vi "Rinocloud_real-time_monitoring.vi"() -> ()   [LabVIEW 2011, in "Rinocloud Library.lvlib"]
uses:
  Rinocloud Library.lvlib
  Rinocloud_global_variable.vi
  Rinocloud API endpoint VIs/API_endpoint_subVIs/Rinocloud_get_metadata_field_value_subVIs/get_string_value.vi
  Rinocloud API endpoint VIs/API_endpoint_subVIs/Rinocloud_get_metadata_field_value_subVIs/get_numeric_value.vi
panel:
  out "Local status:":string="OFF"
  in  "Toggle":bool
  out "Sending...":bool
  out "System Waveform Graph":dbl[](graph)
  out "Data chunk":string
  in  "Record name":string
  in  "create empty":bool
  in  "Request period (s)":dbl=1.0 format="%#.2f"
  out "Remote status:":string="OFF"
  in  "stop":bool
  out "Parent folder:":string
  # "Request period and measurement status\ncan be set remotely by\n{\"period\":<value in s>, \"status\":\"on<or off>\"}\n\nLocal changes of period or/and status are \nupdated immediatelly on Rinocloud."
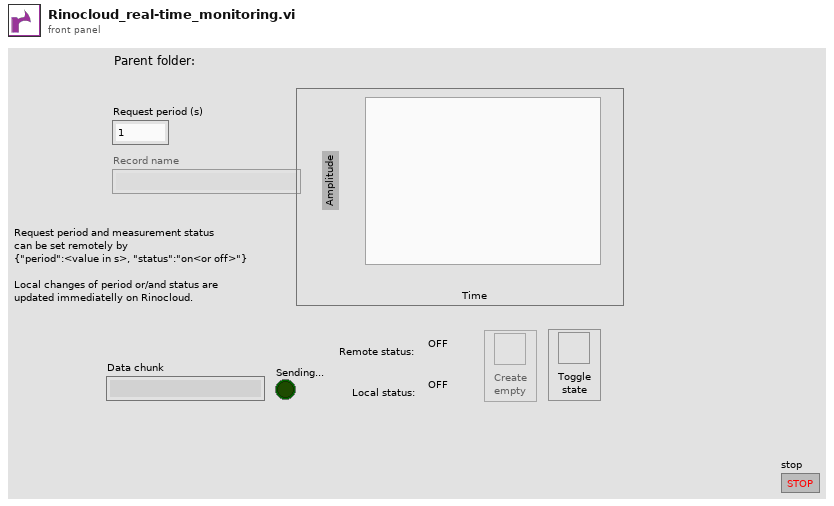
[diagram p1: front panel]
types:
  T1 = cluster{"Record ID":string, "Status":string, "Record name":string, "Parent ID":string, "Request period (s)":dbl, "Sending...":bool, "Parent folder":string, "HTTP resp body":string, "Data chunk":string, "error out":errorcluster, "error in (no error)":errorcluster, "x":dbl, "y array":dbl[], "y":dbl}
  T2 = enum16{"initialize", "create empty", "append", "wait for event", "start append", "generate data"}
  T3 = enum8{"Enabled", "Disabled", "Disabled and Grayed Out"}
  T4 = enum16{"initialize", "create empty", "append", "wait for event"}
  T5 = cluster{"Attribute":string, "Value":string, "Data type":enum16{"Numeric", "String", "1D array of strings", "1D array of doubles", "Data JSON string", "<null>"}}
  T6 = enum16{"Numeric", "String", "1D array of strings", "1D array of doubles", "Data JSON string", "<null>"}
  T7 = cluster{"Attribute":string, "Value":string, "Data type":enum16{"Numeric", "String", "1D array of strings", "1D array of doubles", "Data JSON string", "<null>"}}[]
  T8 = cluster{"headers":string, "body":string, "ID":string, "Saved":bool}
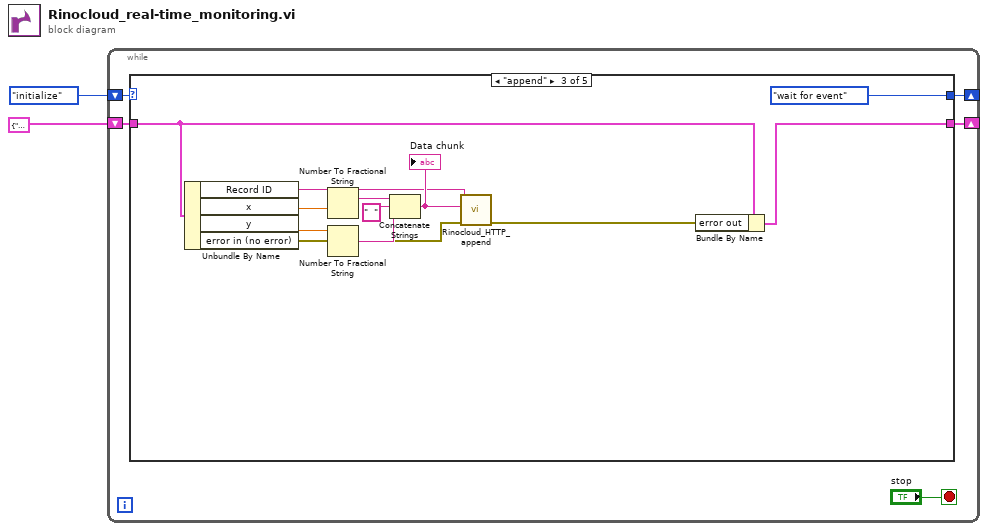
[diagram p0: block diagram]
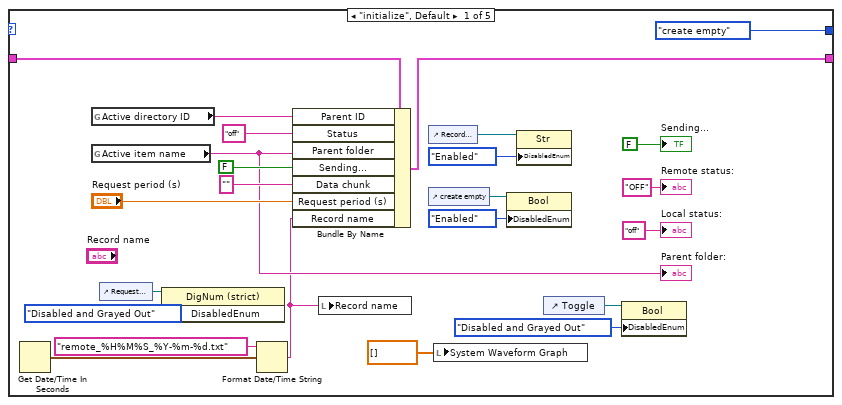
[diagram p2: hidden frame]
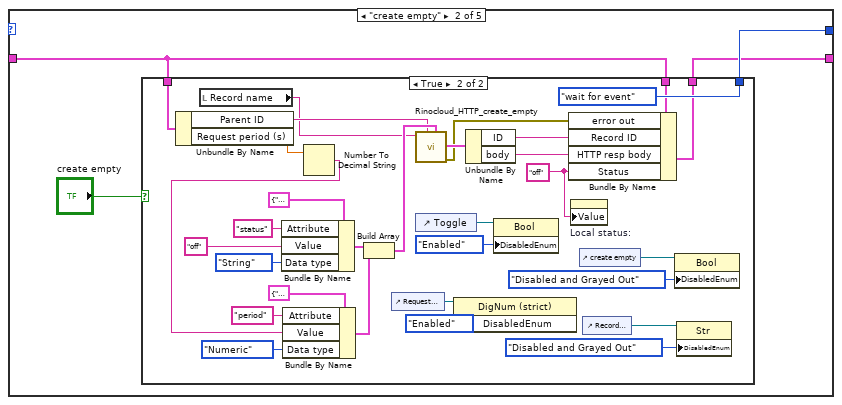
[diagram p3: hidden frame]
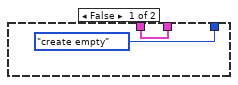
[diagram p4: hidden frame]
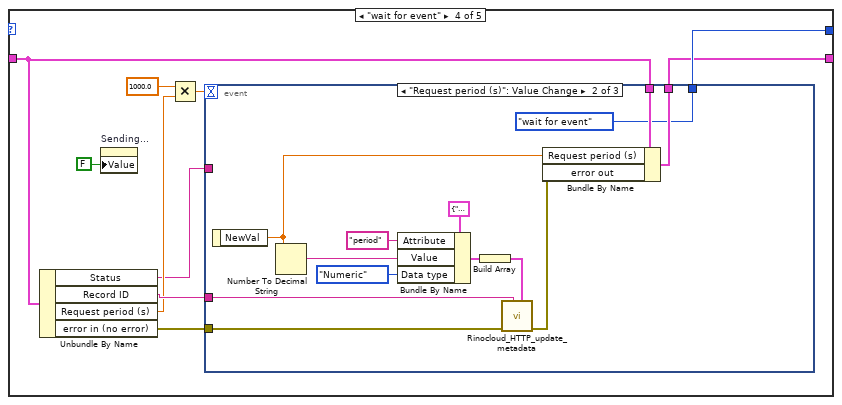
[diagram p5: hidden frame]
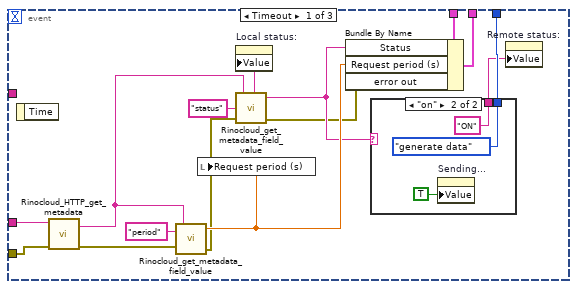
[diagram p6: hidden frame]
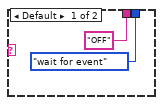
[diagram p7: hidden frame]
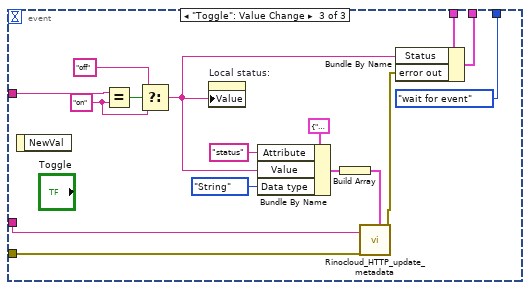
[diagram p8: hidden frame]
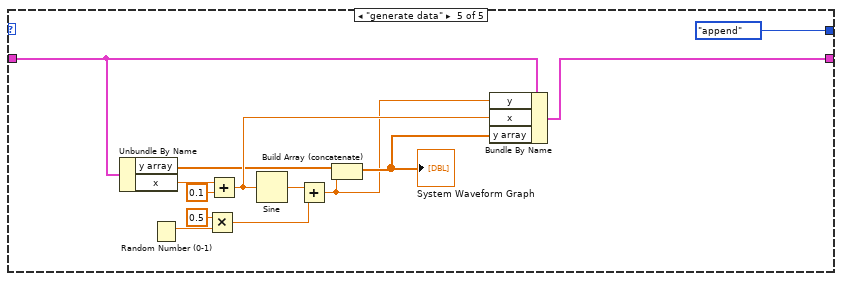
[diagram p9: hidden frame]
diagram:
  n1 = while {
    shift-right: [w3] -> _
    shift-left: T2."initialize" -> [w4]
    shift-right: [w5] -> _
    shift-left: T1 {"Record ID"="", "Status"="", "Record name"="", "Parent ID"="", "Request period (s)"=1.0, "Sending..."=FALSE, "Parent folder"="", "HTTP resp body"="", "Data chunk"="", "error out"={"status"=FALSE, "code"=0, "source"=""}, "error in (no error)"={"status"=FALSE, "code"=0, "source"=""}, "x"=0.0, "y array"=[], "y"=0.0} ("Cluster") -> [w6]
    stop <- "stop" stop-if-true
    n2 = case shown="\"append\"" w4 {
      tunnel: [w30 w32 w69 w84 w141] -> w5
      tunnel: w6 -> [w31 w33 w70 w85 w142]
      tunnel: [T4."create empty" w35 T2."wait for event" w86 T2."append"] -> w3
      frame "initialize", Default {
        n3 = Get Date/Time In Seconds() -> (seconds since 1Jan1904=w14:timestamp)
        n4 = global read "Rinocloud_global_variable.vi" "Active directory ID"() -> (w28:string)
        n5 = global read "Rinocloud_global_variable.vi" "Active item name"() -> (w24:string)
        "Parent folder:" <- w24
        n6 = control-ref of="Request period (s)"() -> (w8:refnum<vi>)
        n7 = property class="DigNum (strict)"(reference=w8, "DisabledEnum"=T3."Disabled and Grayed Out" ("Disabled")) -> ()  [unwired: 1 in, 2 out]
        n8 = Format Date/Time String(time format string (%c)="remote_%H%M%S_%Y-%m-%d.txt", seconds (now)=w14) -> (date/time string=w12:string)  [unwired: 1 in]
        n9 = Bundle By Name(cluster=w31, "Parent ID"=w28, "Status"="off", "Parent folder"=w24, "Sending..."=FALSE, "Data chunk"="", "Request period (s)"="Request period (s)", "Record name"=w12) -> (w30:T1)
        n10 = local write "Record name"(w12) -> ()
        n11 = control-ref of="Record name"() -> (w15:refnum<vi>)
        n12 = control-ref of="create empty"() -> (w22:refnum<vi>)
        n13 = local write "System Waveform Graph"(dbl[] [] ("y array")) -> ()
        n14 = property class="Bool"(reference=w22, "DisabledEnum"=T3."Enabled" ("Disabled")) -> ()  [unwired: 1 in, 2 out]
        n15 = property class="Str"(reference=w15, "DisabledEnum"=T3."Enabled" ("Disabled")) -> ()  [unwired: 1 in, 2 out]
        n16 = control-ref of="Toggle"() -> (w10:refnum<vi>)
        n17 = property class="Bool"(reference=w10, "DisabledEnum"=T3."Disabled and Grayed Out" ("Disabled")) -> ()  [unwired: 1 in, 2 out]
        "Remote status:" <- "OFF" ("Status:")
        "Sending..." <- FALSE ("Sending...")
        "Local status:" <- "off" ("Status:")
      }
      frame "create empty" {
        n18 = case shown="True" "create empty" {
          tunnel: [T4."create empty" T4."wait for event"] -> w35
          tunnel: w33 -> [_ w60]
          tunnel: w33 -> [w36 w58]
          tunnel: [w36 w57] -> w32
          frame False {
          }
          frame True {
            w46 = "off" ("Status:")
            n19 = Unbundle By Name(w60) -> ("Parent ID"=w59:string, "Request period (s)"=w49:dbl)
            n20 = local read "Record name"() -> (w43:string)
            n21 = Bundle By Name(cluster=T5 {"Attribute"="", "Value"="", "Data type"=enum."<null>"} ("extra information field 4"), "Attribute"="status", "Value"="off", "Data type"=T6."String") -> (w64:T5)
            n22 = Number To Decimal String(number=w49) -> (decimal integer string=w48:string)  [unwired: 1 in]
            n23 = Bundle By Name(cluster=T5 {"Attribute"="", "Value"="", "Data type"=enum."<null>"} ("extra information field 4"), "Attribute"="period", "Value"=w48, "Data type"=T6."Numeric") -> (w47:T5)
            n24 = Build Array(w64, w47) -> (w63:T7)
            n25 = control-ref of="Request period (s)"() -> (w39:refnum<vi>)
            n26 = call "Rinocloud_HTTP_create_empty.vi"("Extra metadata array"=w63, "Parent ID"=w59, "Name"=w43) -> ("error out"=w38:errorcluster, "Status"=w62:T8)  [unwired: 5 in]
            n27 = control-ref of="Toggle"() -> (w41:refnum<vi>)
            n28 = property class="DigNum (strict)"(reference=w39, "DisabledEnum"=T3."Enabled" ("Disabled")) -> ()  [unwired: 1 in, 2 out]
            n29 = Unbundle By Name(w62) -> ("ID"=w56:string, "body"=w55:string)
            n30 = property class="Bool"(reference=w41, "DisabledEnum"=T3."Enabled" ("Disabled")) -> ()  [unwired: 1 in, 2 out]
            n31 = Bundle By Name(cluster=w58, "error out"=w38, "Record ID"=w56, "HTTP resp body"=w55, "Status"=w46) -> (w57:T1)
            n32 = property on="Local status:" class="Str"("Value"=w46) -> ()  [unwired: 2 in, 2 out]
            n33 = control-ref of="create empty"() -> (w54:refnum<vi>)
            n34 = control-ref of="Record name"() -> (w45:refnum<vi>)
            n35 = property class="Bool"(reference=w54, "DisabledEnum"=T3."Disabled and Grayed Out" ("Disabled")) -> ()  [unwired: 1 in, 2 out]
            n36 = property class="Str"(reference=w45, "DisabledEnum"=T3."Disabled and Grayed Out" ("Disabled")) -> ()  [unwired: 1 in, 2 out]
          }
        }
      }
      frame "append" {
        n37 = Unbundle By Name(w70) -> ("Record ID"=w75:string, "x"=w76:dbl, "y"=w74:dbl, "error in (no error)"=w72:errorcluster)
        n38 = Number To Fractional String(number=w76) -> (F-format string=w78:string)  [unwired: 3 in]
        n39 = Number To Fractional String(number=w74) -> (F-format string=w80:string)  [unwired: 3 in]
        n40 = Concatenate Strings(w78, "  " ("string"), w80) -> (w77:string)
        "Data chunk" <- w77
        n41 = call "Rinocloud_HTTP_append.vi"("error in (no error)"=w72, "chunk"=w77, "ID"=w75) -> ("error out"=w71:errorcluster)  [unwired: 3 in, 2 out]
        n42 = Bundle By Name(cluster=w70, "error out"=w71) -> (w69:T1)
      }
      frame "wait for event" {
        n43 = Unbundle By Name(w85) -> ("Status"=w83:string, "Record ID"=w90:string, "Request period (s)"=w88:dbl, "error in (no error)"=w81:errorcluster)
        n44 = property on="Sending..." class="Bool (strict)"("Value"=FALSE ("Sending...")) -> ()  [unwired: 2 in, 2 out]
        n45 = Multiply(x=1000.0, y=w88) -> (x*y=w89:dbl)
        n46 = event shown="[1] \"Request period (s)\": Value Change" {
          selector: _ -> [_ _ _]
          dyn-events: _ -> [_ _ _]
          timeout: w89 -> [_ _ _]
          tunnel: w90 -> [w103 w112 w130]
          tunnel: [w102 T2."wait for event" T2."wait for event"] -> w86
          tunnel: w85 -> [w100 w122 w128]
          tunnel: [w99 w121 w127] -> w84
          tunnel: w83 -> [_ _ w138]
          tunnel: w81 -> [w94 w111 w123]
          event Timeout {
            n47 = event-data() -> ()  [unwired: 1 in, 1 out]
            n48 = call "Rinocloud_HTTP_get_metadata.vi"("error in (no error)"=w94, "id"=w103) -> ("error out"=w93:errorcluster, "metadata (JSON)"=w95:string)  [unwired: 3 in, 5 out]
            n49 = call-poly "Rinocloud_get_metadata_field_value.vi"("error in (no error)"=w93, "field name"="period", "metadata JSON string"=w95) -> ("error out"=w92:errorcluster, "field value"=w97:dbl)  [unwired: 1 in]
            n50 = local write "Request period (s)"(w97) -> ()
            n51 = call-poly "Rinocloud_get_metadata_field_value.vi"("error in (no error)"=w92, "field name"="status" ("Parameter Name"), "metadata JSON string"=w95) -> ("error out"=w91:errorcluster, "field value"=w96:string)  [unwired: 1 in]
            n52 = property on="Local status:" class="Str"("Value"=w96) -> ()  [unwired: 2 in, 2 out]
            n53 = Bundle By Name(cluster=w100, "Status"=w96, "Request period (s)"=w97, "error out"=w91) -> (w99:T1)
            n54 = case shown="\"on\"" w96 {
              tunnel: [T2."wait for event" T2."generate data"] -> w102
              tunnel: ["OFF" ("Parameter Name") "ON" ("Parameter Name")] -> w101
              frame Default {
              }
              frame "on" {
                n55 = property on="Sending..." class="Bool (strict)"("Value"=TRUE ("Sending...")) -> ()  [unwired: 2 in, 2 out]
              }
            }
            n56 = property on="Remote status:" class="Str"("Value"=w101) -> ()  [unwired: 2 in, 2 out]
          }
          event "Request period (s)": Value Change {
            n57 = event-data() -> ("NewVal"=w115:dbl)  [unwired: 1 in]
            n58 = Number To Decimal String(number=w115) -> (decimal integer string=w116:string)  [unwired: 1 in]
            n59 = Bundle By Name(cluster=T5 {"Attribute"="", "Value"="", "Data type"=enum."<null>"} ("extra information field 4"), "Attribute"="period", "Value"=w116, "Data type"=T6."Numeric") -> (w114:T5)
            n60 = Build Array(w114) -> (w113:T7)
            n61 = call "Rinocloud_HTTP_update_metadata.vi"("Extra metadata array"=w113, "self ID"=w112, "error in (no error)"=w111) -> ("error out"=w110:errorcluster)  [unwired: 7 in, 1 out]
            n62 = Bundle By Name(cluster=w122, "Request period (s)"=w115, "error out"=w110) -> (w121:T1)
          }
          event "Toggle": Value Change {
            w126 = "on" ("y")
            n63 = event-data() -> ()  [unwired: 1 in, 1 out]
            n64 = Equal?(x=w138, y=w126) -> (x = y?=w132:bool)
            n65 = Select(t="off" ("y"), s=w132, f=w126) -> (s? t:f=w125:string)
            n66 = property on="Local status:" class="Str"("Value"=w125) -> ()  [unwired: 2 in, 2 out]
            n67 = Bundle By Name(cluster=T5 {"Attribute"="", "Value"="", "Data type"=enum."<null>"} ("extra information field 4"), "Attribute"="status", "Value"=w125, "Data type"=T6."String") -> (w134:T5)
            n68 = Build Array(w134) -> (w133:T7)
            n69 = call "Rinocloud_HTTP_update_metadata.vi"("Extra metadata array"=w133, "self ID"=w130, "error in (no error)"=w123) -> ("error out"=w124:errorcluster)  [unwired: 7 in, 1 out]
            n70 = Bundle By Name(cluster=w128, "Status"=w125, "error out"=w124) -> (w127:T1)
          }
        }
      }
      frame "generate data" {
        n71 = Unbundle By Name(w142) -> ("y array"=w144:dbl[], "x"=w143:dbl)
        n72 = Random Number (0-1)() -> (number: 0 to 1=w150:dbl)
        n73 = Multiply(x=0.5, y=w150) -> (x*y=w147:dbl)
        n74 = Add(x=w143, y=0.1) -> (x+y=w146:dbl)
        n75 = Sine(x=w146) -> (sin(x)=w148:dbl)
        n76 = Add(x=w148, y=w147) -> (x+y=w140:dbl)
        n77 = Build Array (concatenate)(w144, w140) -> (w145:dbl[])
        "System Waveform Graph" <- w145
        n78 = Bundle By Name(cluster=w142, "y"=w140, "x"=w146, "y array"=w145) -> (w141:T1)
      }
    }
  }
